vi "Initialize.vi"(7 "Channel Name":string="Setpoint.ch%d.SP", 8 "error in":errorcluster, 9 "Number of Channels":u32=1, 10 "Instance Name":string="PluginName", 11 "Humidity Setpoint in":refnum<class "Humidity Setpoint.lvclass">) -> (0 "error out":errorcluster, 3 "Humidity Setpoint out":refnum<class "Humidity Setpoint.lvclass">)   [LabVIEW 2023, in "Humidity Setpoint.lvclass"]
uses:
  Humidity Setpoint.lvclass
  Humidity Setpoint.lvclass/Humidity Setpoint.ctl
  Parents/Setpoint/Setpoint.lvclass
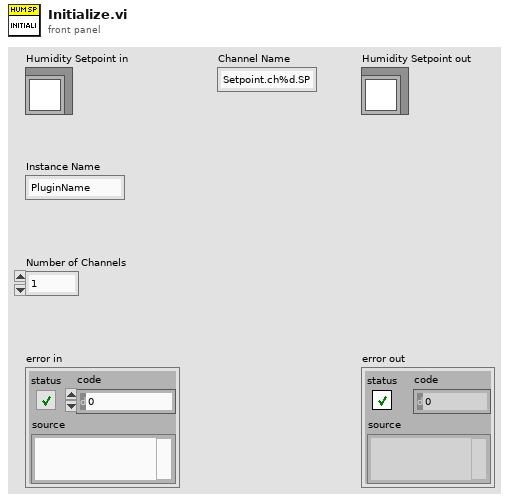
[diagram p1: front panel]
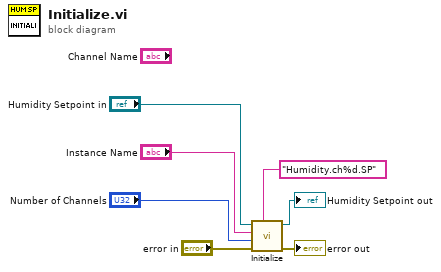
[diagram p0: block diagram]
diagram:
  n1 = call-parent "Initialize.vi"("Channel Name"="Humidity.ch%d.SP", "error in"="error in", "Number of Channels"="Number of Channels", "Instance Name"="Instance Name", "Setpoint in"="Humidity Setpoint in") -> ("error out"=→"error out":errorcluster, "Setpoint out"=→"Humidity Setpoint out":refnum<class "Humidity Setpoint.lvclass">)  [unwired: 5 in]
